vi "Ref_Num_Calibrate_Open.vi"(1 "Test Failed":refnum<vi>, 3 "Open Calibration Successful":refnum<vi>, 8 "error in":errorcluster, 9 "Stop Test":refnum<vi>, 10 "LowCapMode?":refnum<vi>, 11 "Calibration Test":refnum<vi>) -> (0 "error out":errorcluster)   [LabVIEW 2020]
uses:
  <vilib>/Utility/error.llb/DialogType.ctl
  Global 1.vi
panel:
  out "Test Failed LED":bool
  in  "error in 2":errorcluster
  out "Value_TSV":dbl
  out "Meas_TSV":string
  out "Read_TSV":string
  out "serial poll byte 3rd":i16
  out "serial poll byte 1st":i16
  out "LowCapMode?":bool
  out "message":string=" INSTRUCTIONS:\r\rNormal Use:  When using subVIs that incorporate the error in/error out (or error I/O) structure, place this handler where you want to inform the user of an error, typically at the end of the I/O data path, as the last action of the program.  If the error in error? is ERROR, the handler creates a message describing the error and its source.  If the type of dialog = 1 (default), the message is displayed to the user, who can only acknowedge it.  If the type = 2, the user can acknowledge the message or abort execution; aborting a program with active I/O is not recommended.  If the type = 0, no message is displayed; this is used to process the error programmatically, and the error out cluster elements are wired to individual terminals for that reason.  \r\rOther Use:\n\r\nlocal testing.  To test the error code of a subVI or function that does not have the error I/O structure, you can wire its error code and a source string to the local error code and error source inputs.  If error in error? indicates no error and error code is not equal to 0, the local code and source are substituted for the error in values, and error? is set TRUE (ERROR)."
  in  "Cal_Delay_Step":u16
  out "serial poll byte 2nd":i16
  out "Failed Test Count":i32
  out "Test Count":i32
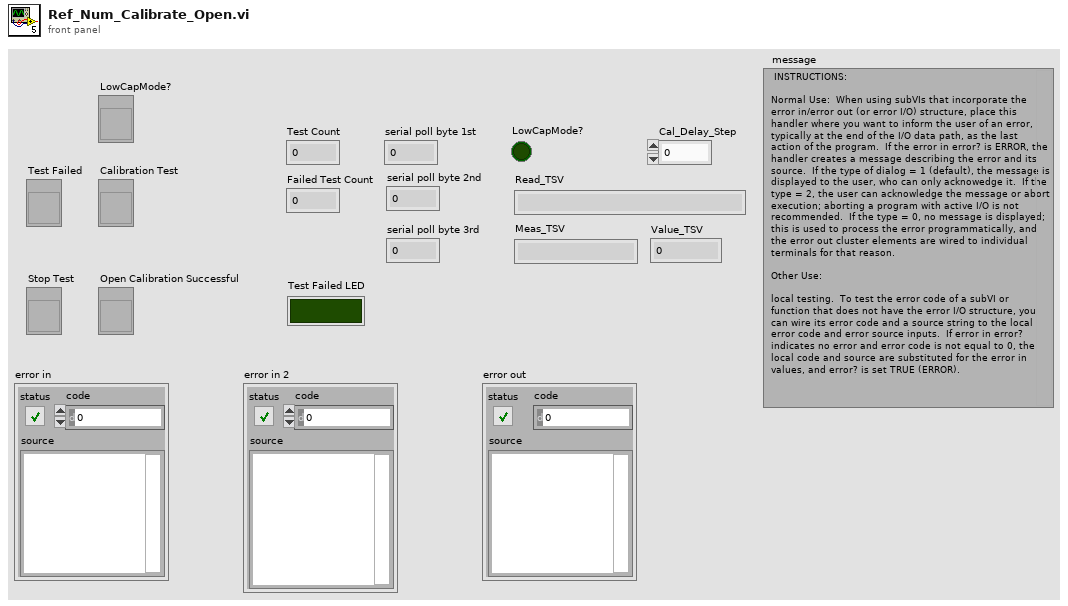
[diagram p1: front panel]
types:
  T1 = typedef "DialogType.ctl" = u16
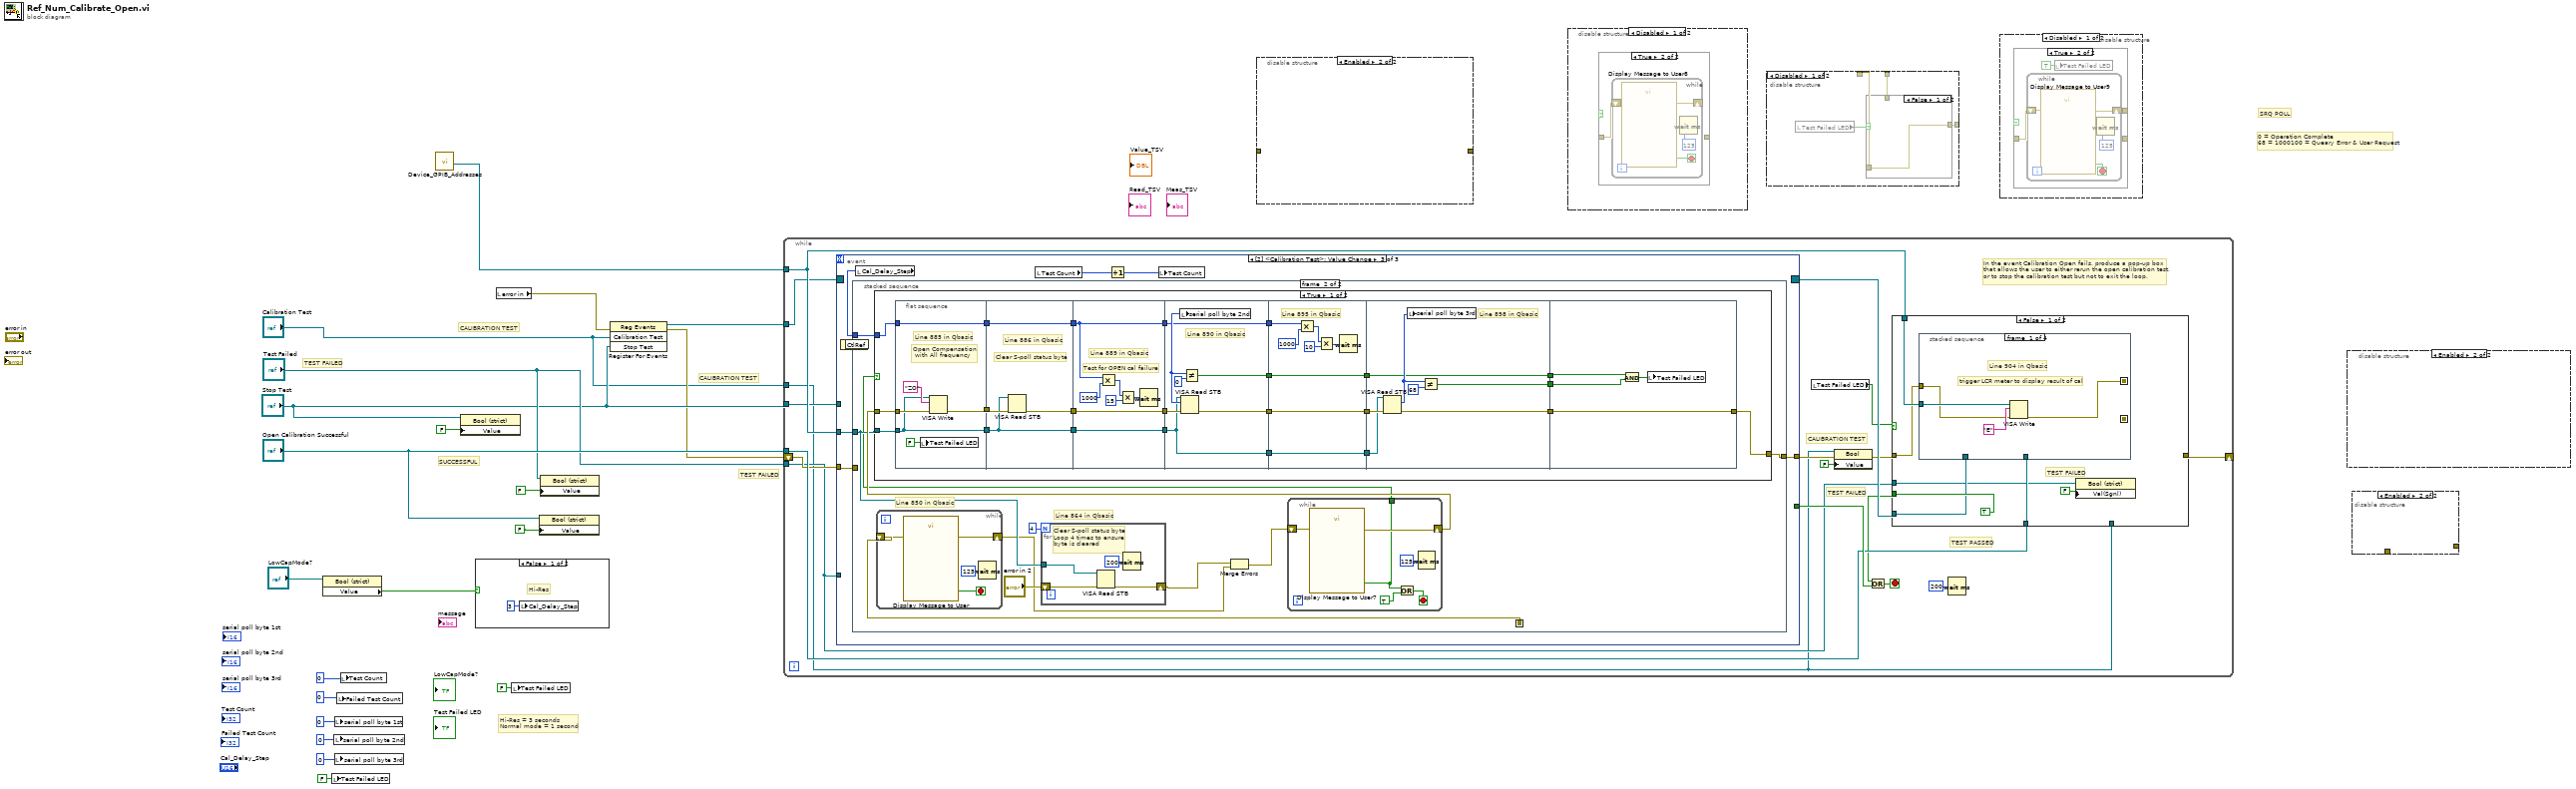
[diagram p0: block diagram]
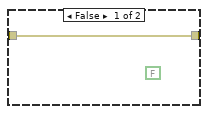
[diagram p6: hidden frame]
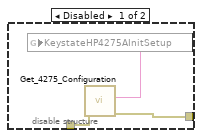
[diagram p8: hidden frame]
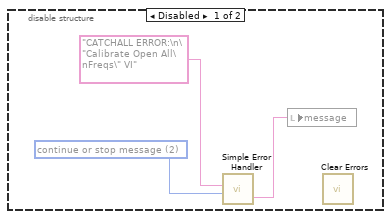
[diagram p9: hidden frame]
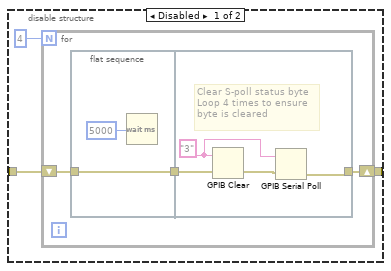
[diagram p10: hidden frame]
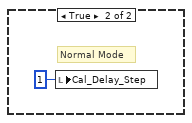
[diagram p11: hidden frame]
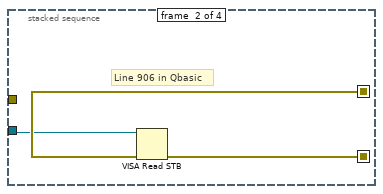
[diagram p12: hidden frame]
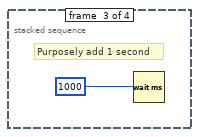
[diagram p13: hidden frame]
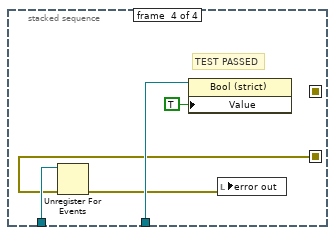
[diagram p14: hidden frame]
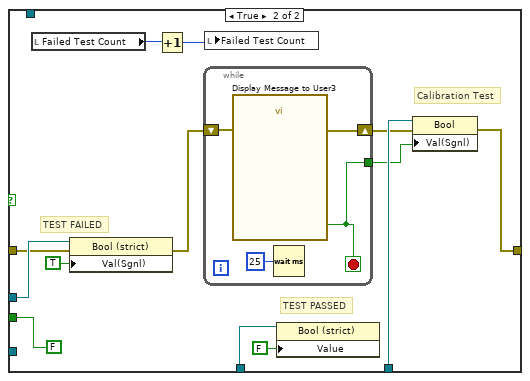
[diagram p15: hidden frame]
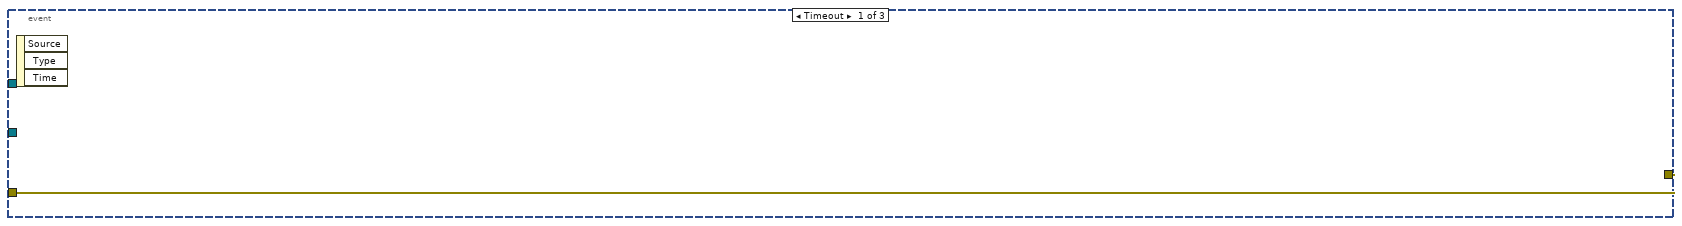
[diagram p16: hidden frame]
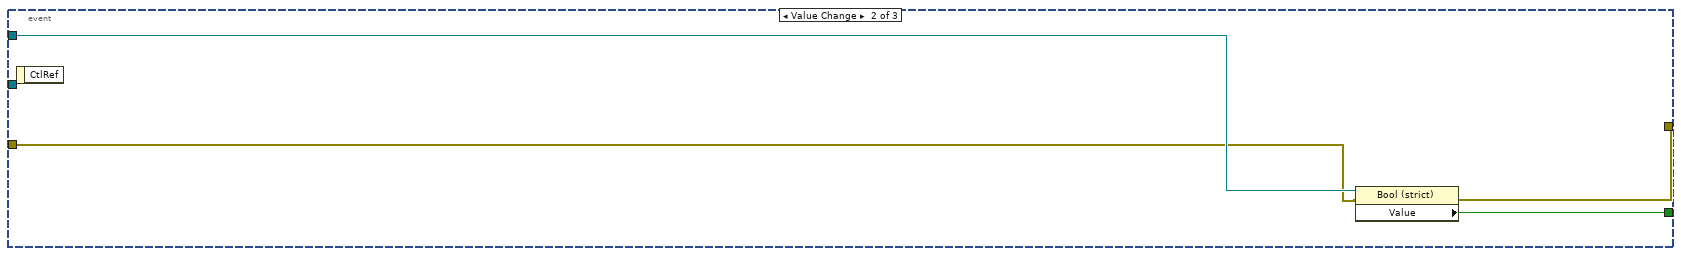
[diagram p17: hidden frame]
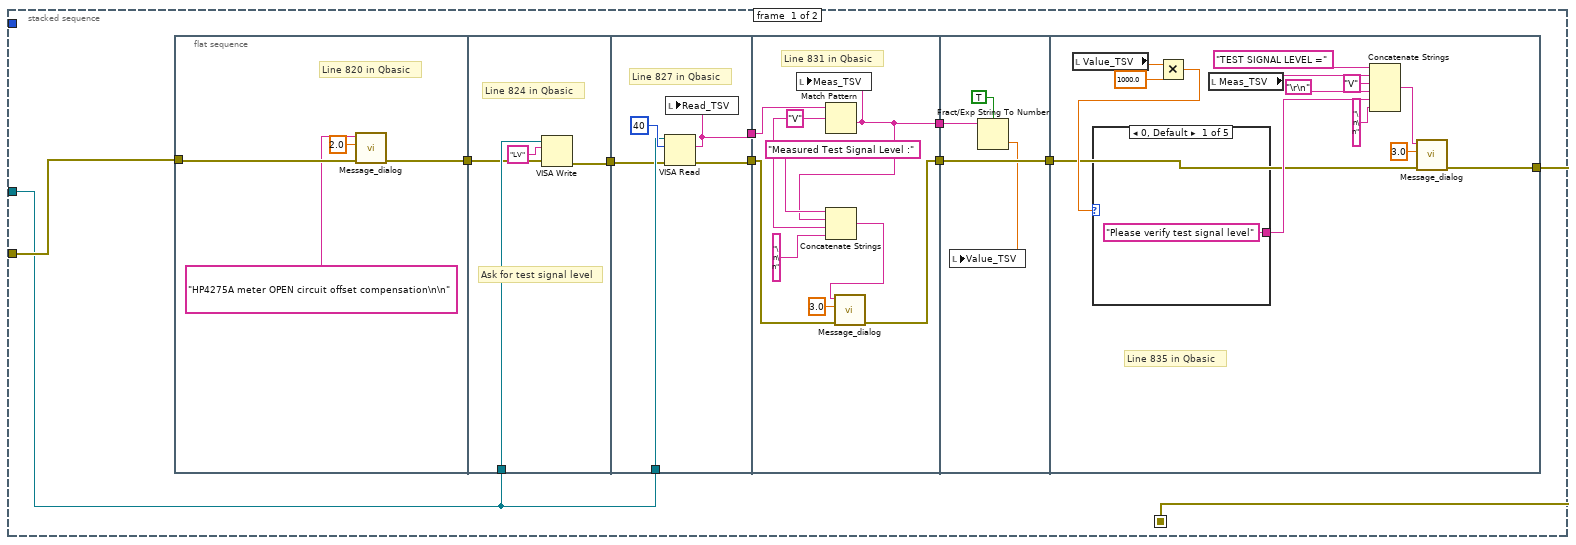
[diagram p18: hidden frame]
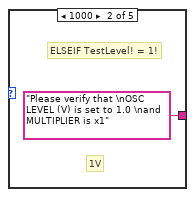
[diagram p19: hidden frame]
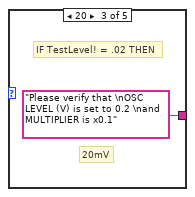
[diagram p20: hidden frame]
diagram:
  # "CALIBRATION TEST"
  # "TEST FAILED"
  # "CALIBRATION TEST"
  # "TEST FAILED"
  # "0 = Operation Complete\n68 = 1000100 = Queary Error & User Request"
  # "SRQ POLL"
  # "SUCCESSFUL"
  # "Hi-Res = 3 seconds\nNormal mode = 1 second"
  n1 = property class="Bool (strict)"(reference="LowCapMode?") -> ("Value"=w14:bool)  [unwired: 1 in, 2 out]
  n2 = local write "Test Failed LED"(FALSE ("Test Failed LED")) -> ()
  n3 = local write "serial poll byte 2nd"(i16 0 ("serial poll byte")) -> ()
  n4 = local write "serial poll byte 1st"(i16 0 ("serial poll byte")) -> ()
  n5 = local write "serial poll byte 3rd"(i16 0 ("serial poll byte")) -> ()
  n6 = local write "Failed Test Count"(0 ("Failed Test Count")) -> ()
  n7 = local write "Test Count"(0 ("Numeric")) -> ()
  n8 = call "Device_GPIB_Addresses.vi"() -> ("HP 4275A Address"=w20:refnum<visa-resource-name>)  [unwired: 9 in, 2 out]
  n9 = property class="Bool (strict)"(reference="Stop Test", "Value"=FALSE ("Test Failed")) -> ()  [unwired: 1 in, 2 out]
  n10 = case shown="False" w14 {
    frame False {
      # "Hi-Res"
      n11 = local write "Cal_Delay_Step"(u16 3 ("Cal_Delay_Step")) -> ()
    }
    frame True {
      # "Normal Mode"
      n12 = local write "Cal_Delay_Step"(u16 1 ("Cal_Delay_Step")) -> ()
    }
  }
  n13 = local read "error in"() -> (w6:errorcluster)
  n14 = local write "Test Failed LED"(FALSE ("Test Failed LED")) -> ()
  n15 = property class="Bool (strict)"(reference="Open Calibration Successful", "Value"=FALSE ("Open Calibration Successful")) -> ()  [unwired: 1 in, 2 out]
  n16 = property class="Bool (strict)"(reference="Test Failed", "Value"=FALSE ("Test Failed")) -> ()  [unwired: 1 in, 2 out]
  n17 = register-events(error in=w6, "Calibration Test", "Stop Test") -> (reference out=w5:refnum<event-registration>, error out=w4:errorcluster)  [unwired: 1 in]
  n18 = while {
    tunnel: w20 -> [w36]
    tunnel: "Calibration Test" -> [w23]
    tunnel: "Open Calibration Successful" -> [w35]
    tunnel: "Test Failed" -> [w30]
    shift-right: [w29] -> _
    shift-left: w4 -> [w32]
    tunnel: "Stop Test" -> [w34]
    tunnel: w5 -> [w33]
    stop <- w38 stop-if-true
    # "CALIBRATION TEST"
    # "In the event Calibration Open fails, produce a pop-up box\nthat allows the user to either rerun the open calibration test,\nor to stop the calibration test but not to exit the loop."
    # "TEST PASSED"
    # "TEST FAILED"
    n19 = event shown="[2] <Calibration Test>: Value Change" {
      selector: w33 -> [_ _ _]
      dyn-events: [_ _ _] -> w31
      timeout: _ -> [_ _ _]
      tunnel: [_ w81 _] -> w39
      tunnel: w36 -> [_ _ w85]
      tunnel: w32 -> [w77 w79 w84]
      tunnel: w34 -> [_ w80 _]
      tunnel: w30 -> [_ _ _]
      tunnel: [w77 w78 w82] -> w25
      event Timeout {
        n20 = event-data() -> ()  [unwired: 1 in, 3 out]
      }
      event Value Change {
        n21 = event-data() -> ()  [unwired: 1 in, 1 out]
        n22 = property class="Bool (strict)"(reference=w80, error in=w79) -> (error out=w78:errorcluster, "Value"=w81:bool)  [unwired: 1 out]
      }
      event Value Change {
        n23 = event-data() -> ()  [unwired: 1 in, 1 out]
        n24 = local read "Cal_Delay_Step"() -> (w83:u16)
        n25 = stacked-sequence {
          seq-local: [w97 _] -> [_ w149]
          tunnel: w84 -> [w96 _]
          tunnel: w83 -> [_ w152]
          tunnel: w85 -> [w88 w147]
          tunnel: [_ w142] -> w82
          frame #0 {
            n26 = flat-sequence {
              tunnel: w96 -> [w101]
              tunnel: [w100] -> w95
              tunnel: w95 -> [w103]
              tunnel: w88 -> [w104]
              tunnel: [w102] -> w94
              tunnel: w94 -> [w108]
              tunnel: w88 -> [w109]
              tunnel: [w107] -> w93
              tunnel: [w106] -> w92
              tunnel: w93 -> [w114]
              tunnel: w92 -> [w116]
              tunnel: [w113] -> w91
              tunnel: [w118] -> w90
              tunnel: w91 -> [w123]
              tunnel: w90 -> [w122]
              tunnel: [w123] -> w89
              tunnel: [w126] -> w97
              tunnel: w89 -> [w127]
              frame #0 {
                # "Line 820 in Qbasic"
                n27 = call "Message_dialog.vi"("error in (no error)"=w101, "set delay"=2.0, "String"="HP4275A meter OPEN circuit offset compensation\n\n") -> ("error out"=w100:errorcluster)  [unwired: 8 in]
              }
              frame #1 {
                # "Ask for test signal level"
                # "Line 824 in Qbasic"
                n28 = VISA Write(VISA resource name=w104, write buffer="LV" ("data"), error in (no error)=w103) -> (error out=w102:errorcluster)  [unwired: 2 out]
              }
              frame #2 {
                # "Line 827 in Qbasic"
                n29 = VISA Read(VISA resource name=w109, byte count=u32 40, error in (no error)=w108) -> (read buffer=w106:string, error out=w107:errorcluster)  [unwired: 2 out]
                n30 = local write "Read_TSV"(w106) -> ()
              }
              frame #3 {
                w117 = "V" ("regular expression")
                # "Line 831 in Qbasic"
                n31 = Match Pattern(string=w116, regular expression=w117) -> (after substring=w118:string)  [unwired: 1 in, 3 out]
                n32 = local write "Meas_TSV"(w118) -> ()
                n33 = Concatenate Strings("Measured Test Signal Level :", w118, w117, "\n\n" ("string")) -> (w112:string)
                n34 = call "Message_dialog.vi"("error in (no error)"=w114, "set delay"=3.0, "String"=w112) -> ("error out"=w113:errorcluster)  [unwired: 8 in]
              }
              frame #4 {
                n35 = Fract/Exp String To Number(use system decimal point (T)=TRUE, string=w122) -> (number=w121:dbl)  [unwired: 2 in, 1 out]
                n36 = local write "Value_TSV"(w121) -> ()
              }
              frame #5 {
                # "Line 835 in Qbasic"
                n37 = local read "Value_TSV"() -> (w136:dbl)
                n38 = Multiply(x=w136, y=1000.0) -> (x*y=w134:dbl)
                n39 = case shown="0, Default" w134 {
                  tunnel: ["Please verify test signal level" "Please verify that \nOSC LEVEL (V) is set to 1.0 \nand MULTIPLIER is x1" "Please verify that \nOSC LEVEL (V) is set to 0.2 \nand MULTIPLIER is x0.1" "Please verify that \nOSC LEVEL (V) is set to 0.15 \nand MULTIPLIER is x0.1" "Please verify that \nOSC LEVEL (V) is set to 1.0 \nand MULTIPLIER is x0.1"] -> w132
                  frame 0, Default {
                  }
                  frame 1000 {
                    # "1V"
                    # "ELSEIF TestLevel! = 1!"
                  }
                  frame 20 {
                    # "20mV"
                    # "IF TestLevel! = .02 THEN"
                  }
                  frame 15 {
                    # "15mV"
                    # "ELSEIF TestLevel! = .015 THEN"
                  }
                  frame 100 {
                    # "100mV"
                    # "ELSEIF TestLevel! = .1"
                  }
                }
                n40 = local read "Meas_TSV"() -> (w130:string)
                n41 = Concatenate Strings("TEST SIGNAL LEVEL =", w130, "V" ("string"), "\r\n", w132, "\n\n" ("string")) -> (w125:string)
                n42 = call "Message_dialog.vi"("error in (no error)"=w127, "set delay"=3.0, "String"=w125) -> ("error out"=w126:errorcluster)  [unwired: 8 in]
              }
            }
          }
          frame #1 {
            # "Line 864 in Qbasic"
            # "Line 850 in Qbasic"
            n43 = while {
              shift-right: [w326] -> w145
              shift-left: w149 -> [w327]
              stop <- w325 stop-if-true
              n44 = call "Display Message to User"("error in (no error)"=w327) -> ("error out"=w326:errorcluster, "OK"=w325:bool)  [unwired: 9 in]
              n45 = Wait (ms)(milliseconds to wait=u32 125) -> ()  [unwired: 1 out]
            }
            n46 = for {
              N: 4 -> [_]
              shift-right: [w321] -> w146
              shift-left: "error in 2" -> [w322]
              tunnel: w147 -> [w320]
              # "Clear S-poll status byte\nLoop 4 times to ensure\nbyte is cleared"
              n47 = VISA Read STB(8:w322, 11:w320) -> (0:w321:errorcluster)  [unwired: 2 out]
              n48 = Wait (ms)(milliseconds to wait=u32 200) -> ()  [unwired: 1 out]
            }
            n49 = Merge Errors(w146, w145) -> (w144:errorcluster)
            n50 = while {
              tunnel: [w155] -> w143
              shift-right: [w158] -> w148
              shift-left: w144 -> [w157]
              stop <- w154 stop-if-true
              n51 = call "Display Message to User7"("error in (no error)"=w157) -> ("error out"=w158:errorcluster, "ALL Frequency"=w155:bool)  [unwired: 9 in]
              n52 = Or(x=w155, y=TRUE) -> (x .or. y?=w154:bool)
              n53 = Wait (ms)(milliseconds to wait=u32 125) -> ()  [unwired: 1 out]
            }
            n54 = case shown="True" w143 {
              tunnel: w147 -> [w177 w228]
              tunnel: w152 -> [w169 w227]
              tunnel: w148 -> [w178 w226]
              tunnel: [w160 w225] -> w142
              frame True {
                n55 = flat-sequence {
                  tunnel: [w185] -> w179
                  tunnel: w178 -> [w186]
                  tunnel: w177 -> [w184]
                  tunnel: [w184] -> w176
                  tunnel: [w183] -> w170
                  tunnel: w169 -> [w183]
                  tunnel: [w190] -> w181
                  tunnel: w179 -> [w191]
                  tunnel: w176 -> [w189]
                  tunnel: [w189] -> w175
                  tunnel: [w188] -> w171
                  tunnel: w170 -> [w188]
                  tunnel: [w198] -> w180
                  tunnel: w181 -> [w198]
                  tunnel: w175 -> [w197]
                  tunnel: [w197] -> w174
                  tunnel: [w192] -> w172
                  tunnel: w171 -> [w192]
                  tunnel: w180 -> [w203]
                  tunnel: w174 -> [w201]
                  tunnel: [w202] -> w173
                  tunnel: w172 -> [w202]
                  tunnel: [w201] -> w166
                  tunnel: [w200] -> w165
                  tunnel: [w199] -> w164
                  tunnel: w173 -> [w212]
                  tunnel: [w207] -> w168
                  tunnel: [w208] -> w167
                  tunnel: w166 -> [w208]
                  tunnel: w165 -> [w207]
                  tunnel: w164 -> [w206]
                  tunnel: [w206] -> w163
                  tunnel: w168 -> [w220]
                  tunnel: w167 -> [w219]
                  tunnel: w163 -> [w216]
                  tunnel: [w216] -> w162
                  tunnel: [w215] -> w161
                  tunnel: [w214] -> w159
                  tunnel: w162 -> [w224]
                  tunnel: w161 -> [w223]
                  tunnel: [w221] -> w160
                  tunnel: w159 -> [w221]
                  frame #0 {
                    # "Line 885 in Qbasic"
                    # "Open Compensation\n with All frequency"
                    n56 = local write "Test Failed LED"(FALSE ("Test Failed LED")) -> ()
                    n57 = VISA Write(VISA resource name=w184, write buffer="ZO" ("data"), error in (no error)=w186) -> (error out=w185:errorcluster)  [unwired: 2 out]
                  }
                  frame #1 {
                    # "Line 886 in Qbasic"
                    # "Clear S-poll status byte"
                    n58 = VISA Read STB(8:w191, 11:w189) -> (0:w190:errorcluster)  [unwired: 2 out]
                  }
                  frame #2 {
                    # "Line 889 in Qbasic"
                    # "Test for OPEN cal failure"
                    n59 = Multiply(x=w192, y=u16 1000) -> (x*y=w195:u16)
                    n60 = Multiply(x=w195, y=u16 15) -> (x*y=w193:u16)
                    n61 = Wait (ms)(milliseconds to wait=w193) -> ()  [unwired: 1 out]
                  }
                  frame #3 {
                    # "Line 890 in Qbasic"
                    n62 = VISA Read STB(8:w203, 11:w201) -> (0:w200:errorcluster, 2:w204:u16)  [unwired: 1 out]
                    n63 = local write "serial poll byte 2nd"(w204) -> ()
                    n64 = Not Equal?(x=w204, y=i16 0) -> (x != y?=w199:bool)
                  }
                  frame #4 {
                    # "Line 895 in Qbasic"
                    n65 = Multiply(x=w212, y=u16 1000) -> (x*y=w211:u16)
                    n66 = Multiply(x=w211, y=u16 10) -> (x*y=w209:u16)
                    n67 = Wait (ms)(milliseconds to wait=w209) -> ()  [unwired: 1 out]
                  }
                  frame #5 {
                    # "Line 898 in Qbasic"
                    n68 = VISA Read STB(8:w220, 11:w219) -> (0:w214:errorcluster, 2:w217:u16)  [unwired: 1 out]
                    n69 = local write "serial poll byte 3rd"(w217) -> ()
                    n70 = Not Equal?(x=w217, y=i16 68) -> (x != y?=w215:bool)
                  }
                  frame #6 {
                    n71 = And(x=w224, y=w223) -> (x .and. y?=w222:bool)
                    n72 = local write "Test Failed LED"(w222) -> ()
                  }
                }
              }
              frame False {
                n73 = flat-sequence {
                  tunnel: w228 -> [w252]
                  tunnel: [w252] -> w247
                  tunnel: [w251] -> w246
                  tunnel: w227 -> [w251]
                  tunnel: [w250] -> w245
                  tunnel: w226 -> [w249]
                  tunnel: [w260] -> w244
                  tunnel: w247 -> [w260]
                  tunnel: w246 -> [w255]
                  tunnel: [w255] -> w243
                  tunnel: [w254] -> w242
                  tunnel: w245 -> [w254]
                  tunnel: [w264] -> w241
                  tunnel: w244 -> [w264]
                  tunnel: [w263] -> w240
                  tunnel: w243 -> [w263]
                  tunnel: w242 -> [w262]
                  tunnel: [w261] -> w239
                  tunnel: [w272] -> w238
                  tunnel: w241 -> [w272]
                  tunnel: w240 -> [w266]
                  tunnel: [w267] -> w237
                  tunnel: w239 -> [w267]
                  tunnel: [w266] -> w236
                  tunnel: w238 -> [w276]
                  tunnel: [w276] -> w235
                  tunnel: w237 -> [w275]
                  tunnel: [w274] -> w234
                  tunnel: [w273] -> w233
                  tunnel: w236 -> [w273]
                  tunnel: w235 -> [w279]
                  tunnel: w234 -> [w282]
                  tunnel: [w281] -> w232
                  tunnel: [w280] -> w231
                  tunnel: [w279] -> w230
                  tunnel: [w278] -> w229
                  tunnel: w233 -> [w278]
                  tunnel: w232 -> [w288]
                  tunnel: w231 -> [w286]
                  tunnel: w230 -> [w285]
                  tunnel: w229 -> [w284]
                  tunnel: [w283] -> w225
                  frame #0 {
                    # "Line 870 in Qbasic"
                    # "Self Test ON \nand STORE"
                    n74 = local write "Test Failed LED"(FALSE ("Test Failed LED")) -> ()
                    n75 = VISA Write(VISA resource name=w252, write buffer="&9" ("data"), error in (no error)=w249) -> (error out=w250:errorcluster)  [unwired: 2 out]
                  }
                  frame #1 {
                    # "Line 871 in Qbasic"
                    n76 = Multiply(x=w255, y=u16 1000) -> (x*y=w257:u16)
                    n77 = Add(x=w257, y=u16 2000) -> (x+y=w258:u16)
                    n78 = Wait (ms)(milliseconds to wait=w258) -> ()  [unwired: 1 out]
                  }
                  frame #2 {
                    # "Line 872 in Qbasic"
                    # "OPEN compensation,\n single freq."
                    n79 = VISA Write(VISA resource name=w264, write buffer="ZO" ("data"), error in (no error)=w262) -> (error out=w261:errorcluster)  [unwired: 2 out]
                  }
                  frame #3 {
                    # "Line 873 in Qbasic"
                    n80 = Multiply(x=w266, y=u16 1000) -> (x*y=w270:u16)
                    n81 = Add(x=w270, y=u16 3000) -> (x+y=w269:u16)
                    n82 = Wait (ms)(milliseconds to wait=w269) -> ()  [unwired: 1 out]
                  }
                  frame #4 {
                    # "Line 874 in Qbasic"
                    # "Self Test OFF"
                    n83 = VISA Write(VISA resource name=w276, write buffer="S0" ("data"), error in (no error)=w275) -> (error out=w274:errorcluster)  [unwired: 2 out]
                  }
                  frame #5 {
                    # "Line 875 in Qbasic"
                    # "Clear S-poll status byte"
                    n84 = VISA Read STB(8:w282, 11:w279) -> (0:w280:errorcluster, 2:w281:u16)  [unwired: 1 out]
                  }
                  frame #6 {
                    # "1st Status Byte"
                    # "Line 876 in Qbasic"
                    n85 = local write "serial poll byte 1st"(w288) -> ()
                    n86 = Not Equal?(x=w288, y=i16 68) -> (x != y?=w287:bool)
                    n87 = case shown="False" w287 {
                      tunnel: w286 -> [w297 w315]
                      tunnel: w285 -> [w296 _]
                      tunnel: w284 -> [w295 _]
                      tunnel: [w290 w313] -> w283
                      frame False {
                        # "Line 880 - 883 in Qbasic"
                        n88 = flat-sequence {
                          tunnel: w297 -> [w301]
                          tunnel: w296 -> [w298]
                          tunnel: [w299] -> w293
                          tunnel: [w298] -> w291
                          tunnel: w295 -> [w306]
                          tunnel: [w304] -> w294
                          tunnel: w293 -> [w304]
                          tunnel: [w302] -> w292
                          tunnel: w291 -> [w302]
                          tunnel: w294 -> [w311]
                          tunnel: w292 -> [w310]
                          tunnel: [w309] -> w290
                          frame #0 {
                            n89 = VISA Write(VISA resource name=w298, write buffer="T1", error in (no error)=w301) -> (error out=w299:errorcluster)  [unwired: 2 out]
                          }
                          frame #1 {
                            n90 = Multiply(x=w306, y=u16 1000) -> (x*y=w303:u16)
                            n91 = Add(x=w303, y=u16 1000) -> (x+y=w308:u16)
                            n92 = Wait (ms)(milliseconds to wait=w308) -> ()  [unwired: 1 out]
                          }
                          frame #2 {
                            n93 = VISA Write(VISA resource name=w310, write buffer="T2", error in (no error)=w311) -> (error out=w309:errorcluster)  [unwired: 2 out]
                          }
                        }
                      }
                      frame True {
                        n94 = local write "Test Failed LED"(TRUE ("Test Failed LED")) -> ()
                        n95 = while {
                          shift-right: [w318] -> w313
                          shift-left: w315 -> [w319]
                          stop <- w317 stop-if-true
                          n96 = call "Display Message to User6"("error in (no error)"=w319) -> ("error out"=w318:errorcluster, "OK"=w317:bool)  [unwired: 9 in]
                          n97 = Wait (ms)(milliseconds to wait=u32 125) -> ()  [unwired: 1 out]
                        }
                      }
                    }
                  }
                }
              }
            }
          }
        }
        n98 = local read "Test Count"() -> (w87:i32)
        n99 = Increment(x=w87) -> (x+1=w86:i32)
        n100 = local write "Test Count"(w86) -> ()
      }
    }
    n101 = local read "Test Failed LED"() -> (w27:bool)
    n102 = property class="Bool"(reference=w23, error in=w25, "Value"=FALSE) -> (error out=w24:errorcluster)  [unwired: 1 out]
    n103 = case shown="False" w27 {
      tunnel: w36 -> [w46 _]
      tunnel: w24 -> [w43 w67]
      tunnel: [TRUE FALSE] -> w28
      tunnel: w35 -> [w44 w61]
      tunnel: w30 -> [w40 w71]
      tunnel: w31 -> [w42 _]
      tunnel: [_ w62] -> w29
      tunnel: w23 -> [_ w65]
      frame False {
        # "TEST FAILED"
        n104 = stacked-sequence {
          seq-local: [w47 _ _ _] -> [_ w53 _ _]
          seq-local: [_ w51 _ _] -> [_ _ _ w55]
          tunnel: w46 -> [w49 w52 _ _]
          tunnel: w44 -> [_ _ _ w59]
          tunnel: w43 -> [w48 _ _ _]
          tunnel: w42 -> [_ _ _ w57]
          frame #0 {
            # "Line 904 in Qbasic"
            # "trigger LCR meter to display result of cal"
            n105 = VISA Write(VISA resource name=w49, write buffer="E" ("data"), error in (no error)=w48) -> (error out=w47:errorcluster)  [unwired: 2 out]
          }
          frame #1 {
            # "Line 906 in Qbasic"
            n106 = VISA Read STB(8:w53, 11:w52) -> (0:w51:errorcluster)  [unwired: 2 out]
          }
          frame #2 {
            # "Purposely add 1 second"
            n107 = Wait (ms)(milliseconds to wait=u16 1000 ("y")) -> ()  [unwired: 1 out]
          }
          frame #3 {
            # "TEST PASSED"
            n108 = Unregister For Events(event registration refnum=w57, error in=w55) -> (error out=w56:errorcluster)
            n109 = property class="Bool (strict)"(reference=w59, "Value"=TRUE) -> ()  [unwired: 1 in, 2 out]
            n110 = local write "error out"(w56) -> ()
          }
        }
        n111 = property class="Bool (strict)"(reference=w40, "Val(Sgnl)"=FALSE ("Value (Signaling)")) -> ()  [unwired: 1 in, 2 out]
      }
      frame True {
        # "TEST PASSED"
        # "Calibration Test"
        # "TEST FAILED"
        n112 = local read "Failed Test Count"() -> (w68:i32)
        n113 = property class="Bool (strict)"(reference=w71, error in=w67, "Val(Sgnl)"=TRUE ("Value (Signaling)")) -> (error out=w66:errorcluster)  [unwired: 1 out]
        n114 = Increment(x=w68) -> (x+1=w69:i32)
        n115 = while {
          tunnel: [w74] -> w64
          shift-right: [w75] -> w63
          shift-left: w66 -> [w76]
          stop <- w74 stop-if-true
          n116 = call "Display Message to User3"("error in (no error)"=w76) -> ("error out"=w75:errorcluster, "OK"=w74:bool)  [unwired: 9 in]
          n117 = Wait (ms)(milliseconds to wait=u32 25) -> ()  [unwired: 1 out]
        }
        n118 = local write "Failed Test Count"(w69) -> ()
        n119 = property class="Bool (strict)"(reference=w61, "Value"=FALSE) -> ()  [unwired: 1 in, 2 out]
        n120 = property class="Bool"(reference=w65, error in=w63, "Val(Sgnl)"=w64) -> (error out=w62:errorcluster)  [unwired: 1 out]
      }
    }
    n121 = Or(x=w28, y=w39) -> (x .or. y?=w38:bool)
    n122 = Wait (ms)(milliseconds to wait=u32 200) -> ()  [unwired: 1 out]
  }
  n123 = disable-structure shown="Enabled" {
    disable-tunnel: _ -> [w329 _]
    disable-tunnel: [w328 _] -> _
    frame Disabled {
      n124 = for {
        N: 4 -> [_]
        shift-right: [w332] -> w328
        shift-left: w329 -> [w333]
        n125 = flat-sequence {
          tunnel: w333 -> [w335]
          tunnel: [w335] -> w331
          tunnel: [w337] -> w332
          tunnel: w331 -> [w339]
          frame #0 {
            n126 = Wait (ms)(milliseconds to wait=u32 5000) -> ()  [unwired: 1 out]
          }
          frame #1 {
            w336 = "3" ("address string")
            # "Clear S-poll status byte\nLoop 4 times to ensure\nbyte is cleared"
            n127 = GPIB Clear(2:w339, 3:w336) -> (0:w338:errorcluster)  [unwired: 1 out]
            n128 = GPIB Serial Poll(0:w336, 1:w338) -> (4:w337:errorcluster)  [unwired: 2 out]
          }
        }
      }
    }
    frame Enabled {
    }
  }
  n129 = disable-structure shown="Disabled" {
    frame Disabled {
      n130 = case shown="True" {
        selector: _ -> [_ _]
        tunnel: _ -> [w341 w342]
        tunnel: [w341 _] -> _
        frame False {
          w340 = FALSE ("OK")
        }
        frame True {
          n131 = while {
            shift-right: [w345] -> _
            shift-left: w342 -> [w346]
            stop <- w344 stop-if-true
            n132 = call "Display Message to User8"("error in (no error)"=w346) -> ("error out"=w345:errorcluster, "OK"=w344:bool)  [unwired: 9 in]
            n133 = Wait (ms)(milliseconds to wait=u32 125) -> ()  [unwired: 1 out]
          }
        }
      }
    }
    frame Enabled {
    }
  }
  n134 = disable-structure shown="Disabled" {
    disable-tunnel: _ -> [w349 _]
    disable-tunnel: [w348 _] -> _
    disable-tunnel: _ -> [w347 _]
    frame Disabled {
      n135 = local read "Test Failed LED"() -> (w350:bool)
      n136 = case shown="False" w350 {
        tunnel: w349 -> [_ w352]
        tunnel: [w351 w352] -> w348
        tunnel: w347 -> [w351 _]
        frame False {
        }
        frame True {
        }
      }
    }
    frame Enabled {
    }
  }
  n137 = disable-structure shown="Disabled" {
    frame Disabled {
      n138 = case shown="True" {
        selector: _ -> [_ _]
        tunnel: _ -> [w353 w354]
        tunnel: [_ w356] -> _
        tunnel: [w353 _] -> _
        frame False {
        }
        frame True {
          n139 = while {
            shift-right: [w359] -> w356
            shift-left: w354 -> [w360]
            stop <- w358 stop-if-true
            n140 = call "Display Message to User9"("error in (no error)"=w360) -> ("error out"=w359:errorcluster, "OK"=w358:bool)  [unwired: 9 in]
            n141 = Wait (ms)(milliseconds to wait=u32 125) -> ()  [unwired: 1 out]
          }
          n142 = local write "Test Failed LED"(TRUE ("Test Failed LED")) -> ()
        }
      }
    }
    frame Enabled {
    }
  }
  n143 = disable-structure shown="Enabled" {
    frame Disabled {
      w362 = T1 2 items=["no dialog", "OK message", "continue or stop message", "OK message + warnings", "continue/stop + warnings"] ("type of dialog (OK msg:1)")
      n144 = call <vilib>:"Simple Error Handler.vi"("error source (\" \")"="CATCHALL ERROR:\n\"Calibrate Open All\nFreqs\" VI" ("error source (\" \")"), "type of dialog (OK msg:1)"=w362) -> ("message"=w361:string)  [unwired: 3 in, 4 out]
      n145 = local write "message"(w361) -> ()
      n146 = call <vilib>:"Clear Errors.vi"() -> ()  [unwired: 6 in, 2 out]
    }
    frame Enabled {
    }
  }
  n147 = disable-structure shown="Enabled" {
    disable-tunnel: _ -> [w365 _]
    disable-tunnel: [w364 _] -> _
    frame Disabled {
      n148 = call "Get_4275_Configuration.vi"("error in"=w365) -> ("error out"=w364:errorcluster, "Keystate"=w366:string)  [unwired: 9 in]
      n149 = global write "Global 1.vi" "KeystateHP4275AInitSetup"(w366) -> ()
    }
    frame Enabled {
    }
  }
